vi "Dialog_Enter Load Setup File Path.vi"(8 "Error In":errorcluster) -> (0 "Error Out":errorcluster, 2 "Cancelled?":bool, 3 "Macro Commands":T1)   [LabVIEW 2012]
doc: "This VI has no controls.\nThis is a dummy whihc runs when user selects a macro command which does not require any arguments"
uses:
  Custom Controls and Typedefs/Macro_CommandStruct.ctl
  Custom Controls and Typedefs/Macro_Action_List.ctl
  Custom Controls and Typedefs/Macro_ArgumentStruct.ctl
panel:
  in  "Cancel Button":bool
  in  "OK Button":bool
  in  "Setup File Path":path
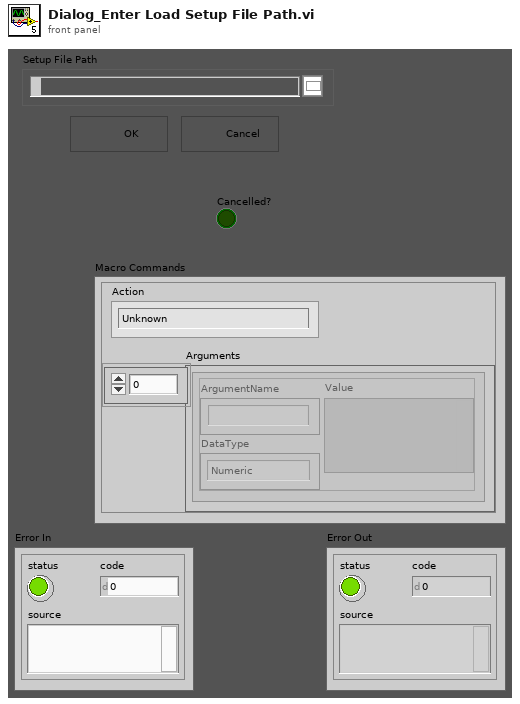
[diagram p1: front panel]
types:
  T1 = typedef "Macro_CommandStruct.ctl" = cluster{"Action":T2, "Arguments":T3[]}
  T2 = typedef "Macro_Action_List.ctl" = enum16{"Unknown", "2D.Frame.Scan", "2D.Line.Scan", "Load.Settings.File", "Move.To.Position", "Pause", "Z.Stack", "LOOP.Start", "LOOP.End"}
  T3 = typedef "Macro_ArgumentStruct.ctl" = cluster{"ArgumentName":string, "DataType":enum16{"Numeric", "String"}, "Value":variant}
  T4 = enum16{"Unknown", "2D.Frame.Scan", "2D.Line.Scan", "Load.Settings.File", "Move.To.Position", "Pause", "Z.Stack", "LOOP.Start", "LOOP.End"}
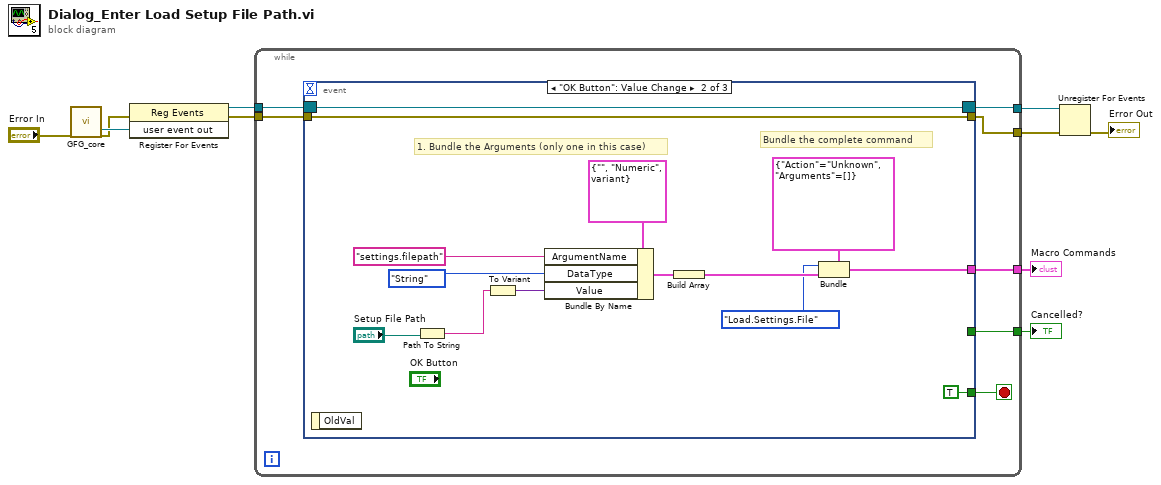
[diagram p0: block diagram]
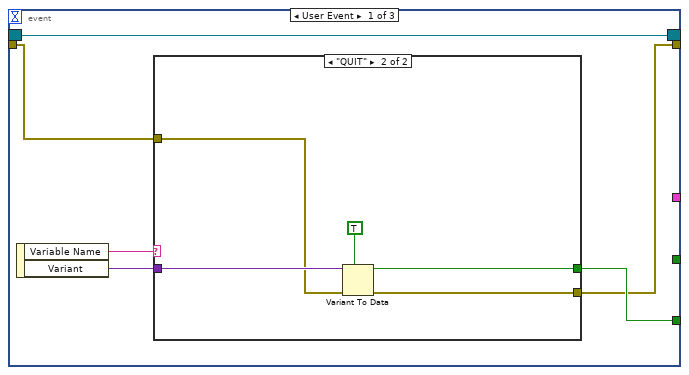
[diagram p2: hidden frame]
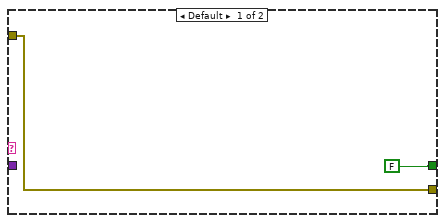
[diagram p3: hidden frame]
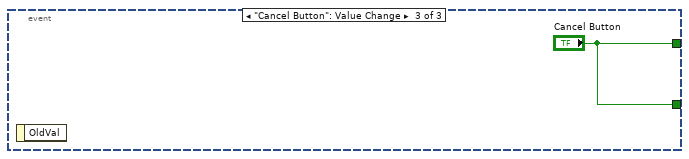
[diagram p4: hidden frame]
diagram:
  n1 = call "GFG_core.vi"("error in (no error)"="Error In") -> ("user event out"=w10:refnum<user-event>, "error out"=w6:errorcluster)  [unwired: 12 in, 5 out]
  n2 = register-events(error in=w6, w10) -> (reference out=w9:refnum<event-registration>, error out=w5:errorcluster)  [unwired: 1 in]
  n3 = while {
    tunnel: w9 -> [w17]
    tunnel: [w16] -> w8
    tunnel: w5 -> [w14]
    tunnel: [w13] -> w4
    tunnel: [w12] -> w3
    tunnel: [w11] -> w1
    stop <- w15 stop-if-true
    n4 = event shown="[1] \"OK Button\": Value Change" {
      selector: w17 -> [w23 w32 _]
      dyn-events: [w23 w32 _] -> w16
      timeout: _ -> [_ _ _]
      tunnel: [w20 TRUE "Cancel Button"] -> w15
      tunnel: w14 -> [w19 w33 _]
      tunnel: [_ w36 _] -> w13
      tunnel: [w18 w33 _] -> w12
      tunnel: [_ _ "Cancel Button"] -> w11
      event User Event {
        n5 = event-data() -> ("Variable Name"=w22:string, "Variant"=w21:variant)  [unwired: 1 in]
        n6 = case shown="\"QUIT\"" w22 {
          tunnel: w21 -> [_ w29]
          tunnel: [FALSE w28] -> w20
          tunnel: w19 -> [w24 w27]
          tunnel: [w24 w26] -> w18
          frame Default {
          }
          frame "QUIT" {
            n7 = Variant To Data(error in=w27, type=TRUE, Variant=w29) -> (data=w28:bool, error out=w26:errorcluster)
          }
        }
      }
      event "OK Button": Value Change {
        # "Bundle the complete command"
        # "1. Bundle the Arguments (only one in this case)"
        n8 = event-data() -> ()  [unwired: 1 in, 1 out]
        n9 = Path To String(path="Setup File Path") -> (string=w34:string)
        n10 = To Variant(anything=w34) -> (Variant=w40:variant)
        n11 = Bundle By Name(cluster=T3 {"ArgumentName"="", "DataType"=enum."Numeric", "Value"=variant} ("Arguments"), "ArgumentName"="settings.filepath", "DataType"=enum16{"Numeric", "String"}."String", "Value"=w40) -> (w39:T3)
        n12 = Build Array(w39) -> (w38:T3[])
        n13 = Bundle(cluster=T1 {"Action"=enum."Unknown", "Arguments"=[]} ("Macro Commands"), "Action"=T4."Load.Settings.File" ("Operation"), "Arguments"=w38) -> (w36:T1)
      }
      event "Cancel Button": Value Change {
        n14 = event-data() -> ()  [unwired: 1 in, 1 out]
      }
    }
  }
  "Macro Commands" <- w4
  "Cancelled?" <- w1
  n15 = Unregister For Events(event registration refnum=w8, error in=w3) -> (error out=→"Error Out":errorcluster)
